vi "操作.vi"(11 "字符串输入":string) -> (3 "字符串输出":string)   [LabVIEW 2016, in "Alarm interface.lvlib"]
uses:
  Alarm interface.lvlib
panel:
  in  "微信":bool
  in  "电话":bool
  in  "短信":bool
  in  "关闭":bool
  in  "确定":bool
  # "操作"
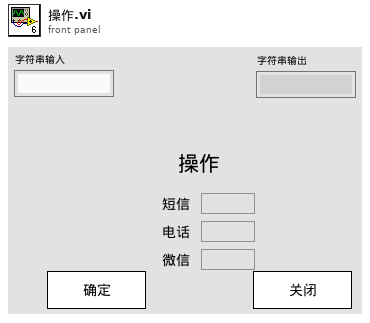
[diagram p1: front panel]
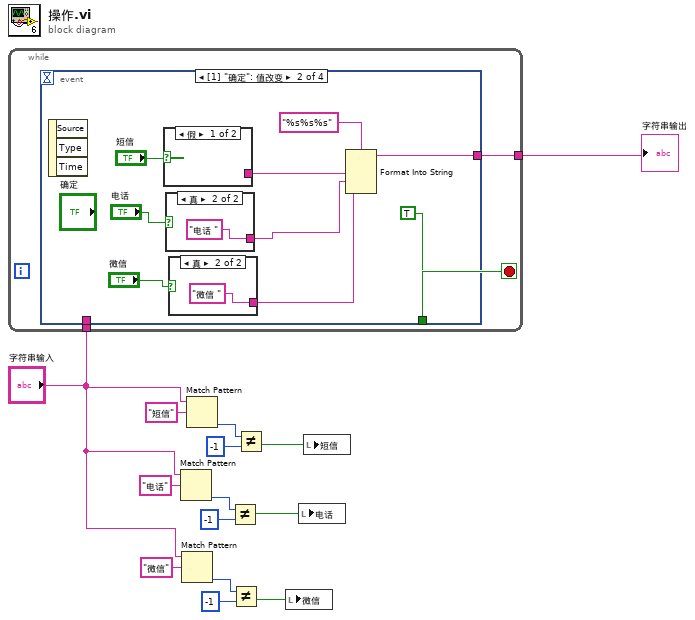
[diagram p0: block diagram]
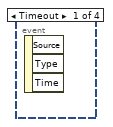
[diagram p2: hidden frame]
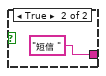
[diagram p5: hidden frame]
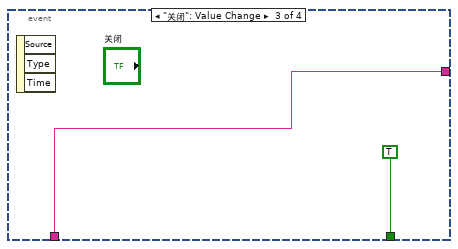
[diagram p6: hidden frame]
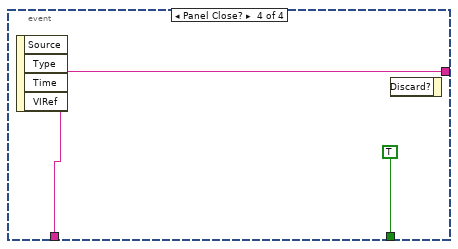
[diagram p7: hidden frame]
diagram:
  n1 = while {
    tunnel: [w16] -> w14
    tunnel: "字符串输入" -> [w15]
    stop <- w17 stop-if-true
    n2 = event shown="[1] \"确定\": 值改变" {
      selector: _ -> [_ _ _ _]
      dyn-events: _ -> [_ _ _ _]
      timeout: _ -> [_ _ _ _]
      tunnel: [_ TRUE TRUE TRUE] -> w17
      tunnel: [_ w24 w30 w32] -> w16
      tunnel: w15 -> [_ _ w30 w32]
      event Timeout {
        n3 = event-data() -> ()  [unwired: 1 in, 3 out]
      }
      event "确定": Value Change {
        n4 = event-data() -> ()  [unwired: 1 in, 3 out]
        n5 = case shown="假" "短信" {
          tunnel: [_ "短信 " ("正则表达式")] -> w22
          frame False {
          }
          frame True {
          }
        }
        n6 = case shown="真" "电话" {
          tunnel: [_ "电话 " ("正则表达式")] -> w20
          frame False {
          }
          frame True {
          }
        }
        n7 = case shown="真" "微信" {
          tunnel: [_ "微信 " ("正则表达式")] -> w18
          frame False {
          }
          frame True {
          }
        }
        n8 = Format Into String(format string="%s%s%s" ("格式字符串"), w22, w20, w18) -> (resulting string=w24:string)  [unwired: 2 in, 1 out]
      }
      event "关闭": Value Change {
        n9 = event-data() -> ()  [unwired: 1 in, 3 out]
      }
      event Panel Close? {
        n10 = event-data() -> ()  [unwired: 1 in, 4 out]
        n11 = event-data() -> ()  [unwired: 2 in, 1 out]
      }
    }
  }
  "字符串输出" <- w14
  n12 = Match Pattern(string="字符串输入", regular expression="电话" ("正则表达式")) -> (offset past match=w8:i32)  [unwired: 1 in, 3 out]
  n13 = Match Pattern(string="字符串输入", regular expression="微信" ("正则表达式")) -> (offset past match=w4:i32)  [unwired: 1 in, 3 out]
  n14 = Match Pattern(string="字符串输入", regular expression="短信" ("正则表达式")) -> (offset past match=w12:i32)  [unwired: 1 in, 3 out]
  n15 = Not Equal?(x=w8, y=-1) -> (x != y?=w6:bool)
  n16 = Not Equal?(x=w4, y=-1) -> (x != y?=w1:bool)
  n17 = Not Equal?(x=w12, y=-1) -> (x != y?=w10:bool)
  n18 = local write "微信"(w1) -> ()
  n19 = local write "电话"(w6) -> ()
  n20 = local write "短信"(w10) -> ()
